vi "SLSC Command Property Node.vi"   [LabVIEW 2020]
doc: "A Property Node with the SLSC Command class preselected. You must open the property using one of the Open Command VIs before you can use SLSC Command Property Node to query information about the command."
uses:
  <resource>/objmgr/slsc.rc
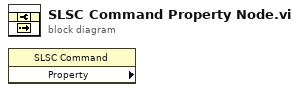
[diagram p0: block diagram]
diagram:
  n1 = property class="SLSC Command" props=[]() -> ()  [unwired: 2 in, 3 out]
